vi "ReadSensors.vi"(8 "error in (no error)":errorcluster, 10 "Sensors":refnum<notifier>, 11 "Refnum in":refnum<k20>) -> (0 "error out":errorcluster, 2 "SettingsAndActuators":T1, 3 "SensorsAndState":T2)   [LabVIEW 2019]
uses:
  Sensors_State.ctl
  Settings_Actuators.ctl
  <vilib>/Utility/error.llb/Error Cluster From Error Code.vi
  <vilib>/rvi/errors/niLvFpgaAdjustHostInterfaceError.vi
  <vilib>/rvi/interface/nirviReadWriteControl/nirviReadWriteControl.xnode
  NiFpgaLv.dll
  <vilib>/rvi/interface/Simulation/niFpgaSimulationCallBeginRW.vi
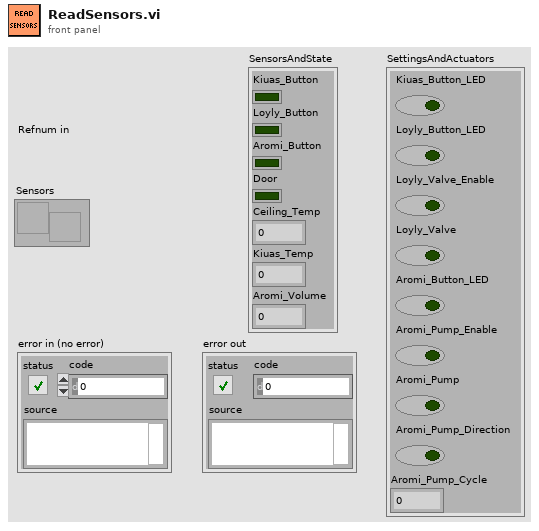
[diagram p1: front panel]
types:
  T1 = typedef "Settings_Actuators.ctl" = cluster{"Kiuas_Button_LED":bool, "Loyly_Button_LED":bool, "Loyly_Valve_Enable":bool, "Loyly_Valve":bool, "Aromi_Button_LED":bool, "Aromi_Pump_Enable":bool, "Aromi_Pump":bool, "Aromi_Pump_Direction":bool, "Aromi_Pump_Cycle":u32}
  T2 = typedef "Sensors_State.ctl" = cluster{"Kiuas_Button":bool, "Loyly_Button":bool, "Aromi_Button":bool, "Door":bool, "Ceiling_Temp":dbl, "Kiuas_Temp":dbl, "Aromi_Volume":dbl}
  T3 = cluster{"Temp0":dbl, "Temp1":dbl, "Vol0":dbl, "Sw0":bool}
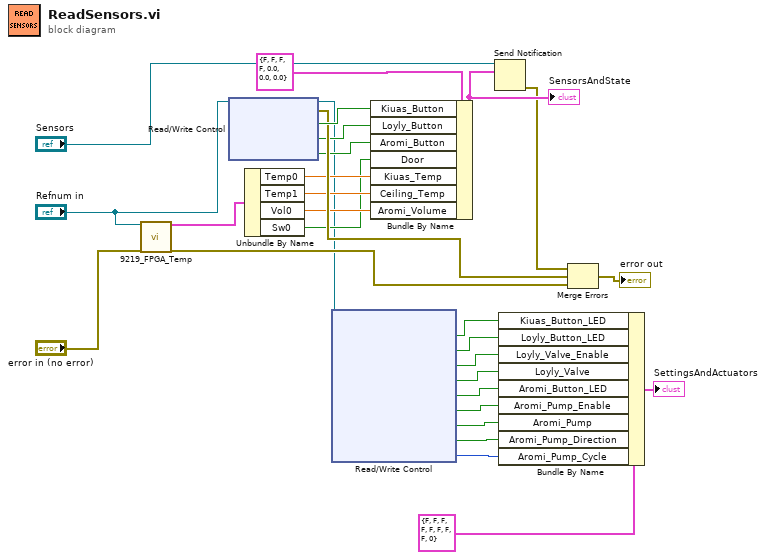
[diagram p0: block diagram]
diagram:
  n1 = call "9219_FPGA_Temp.vi"("FPGA VI Reference"="Refnum in", "error in (no error)"="error in (no error)") -> ("Sensors"=w27:T3, "error out"=w29:errorcluster)  [unwired: 16 in]
  n2 = xnode "Read/Write Control"("FPGA VI Reference In"="Refnum in") -> ("FPGA VI Reference Out"=w13:refnum<k20>, "error out"=w20:errorcluster, "Kiuas Switch"=w21:bool, "Löyly Switch"=w19:bool, "Aromi Switch"=w18:bool)  [unwired: 1 in]
  n3 = Unbundle By Name(w27) -> ("Temp0"=w17:dbl, "Temp1"=w16:dbl, "Vol0"=w15:dbl, "Sw0"=w14:bool)
  n4 = xnode "Read/Write Control"("FPGA VI Reference In"=w13) -> ("Kiuas LED"=w11:bool, "Löyly LED"=w10:bool, "Löyly Valve Enable"=w9:bool, "Löyly Valve"=w8:bool, "Aromi LED"=w7:bool, "Aromi Pump Enable"=w6:bool, "Aromi Pump"=w5:bool, "Pump Direction"=w4:bool, "Pump Cycle"=w3:u32)  [unwired: 1 in, 2 out]
  n5 = Bundle By Name(cluster=T2 {"Kiuas_Button"=FALSE, "Loyly_Button"=FALSE, "Aromi_Button"=FALSE, "Door"=FALSE, "Ceiling_Temp"=0.0, "Kiuas_Temp"=0.0, "Aromi_Volume"=0.0} ("notification"), "Kiuas_Button"=w21, "Loyly_Button"=w19, "Aromi_Button"=w18, "Door"=w14, "Kiuas_Temp"=w17, "Ceiling_Temp"=w16, "Aromi_Volume"=w15) -> (w23:T2)
  "SensorsAndState" <- w23
  n6 = Send Notification(notification=w23, notifier="Sensors") -> (error out=w1:errorcluster)  [unwired: 1 in, 1 out]
  n7 = Bundle By Name(cluster=T1 {"Kiuas_Button_LED"=FALSE, "Loyly_Button_LED"=FALSE, "Loyly_Valve_Enable"=FALSE, "Loyly_Valve"=FALSE, "Aromi_Button_LED"=FALSE, "Aromi_Pump_Enable"=FALSE, "Aromi_Pump"=FALSE, "Aromi_Pump_Direction"=FALSE, "Aromi_Pump_Cycle"=0} ("SettingsActuators"), "Kiuas_Button_LED"=w11, "Loyly_Button_LED"=w10, "Loyly_Valve_Enable"=w9, "Loyly_Valve"=w8, "Aromi_Button_LED"=w7, "Aromi_Pump_Enable"=w6, "Aromi_Pump"=w5, "Aromi_Pump_Direction"=w4, "Aromi_Pump_Cycle"=w3) -> (→"SettingsAndActuators":T1)
  n8 = Merge Errors(w1, w20, w29) -> (→"error out":errorcluster)
